vi "S_curve_scan.vi"() -> ()   [LabVIEW 2017]
panel:
  out "Array 3":dbl[](array[numeric])=[0.064, 0.08600000000000001, 0.10600000000000001, 0.126, 0.14600000000000002, 0.168]
  out "Array 2":dbl[](array[numeric])=[-0.03, -0.04, -0.05, -0.06, -0.07, -0.08]
  out "XY Graph 2":cluster{dbl[], dbl[]}(graph)={[-0.03, -0.04, -0.05, -0.06, -0.07, -0.08], [0.064, 0.08600000000000001, 0.10600000000000001, 0.126, 0.14600000000000002, 0.168]}
  out "time":dbl=10.00580883026123
  out "Current Input":dbl=-0.2
  out "Current DC":dbl=-0.08
  in  "DC end":dbl=-0.08
  in  "DC step":dbl=-0.01
  in  "DC start":dbl=-0.03
  out "Array":dbl[](array[numeric])=[0.05, 0.052000000000000005, 0.054000000000000006, 0.056, 0.058, 0.060000000000000005, 0.062, 0.064, 0.066, 0.068, 0.07, 0.07200000000000001, 0.07400000000000001, 0.07600000000000001, 0.078, 0.08, 0.082, 0.084, 0.08600000000000001, 0.088, 0.09, 0.092, 0.094, 0.096, 0.098, 0.1, 0.10200000000000001, 0.10400000000000001, 0.10600000000000001, 0.10800000000000001, 0.11, 0.112, 0.114, 0.116, 0.11800000000000001, 0.12000000000000001, 0.12200000000000001, 0.124, 0.126, 0.128, 0.13, 0.132, 0.134, 0.136, 0.138, 0.14, 0.14200000000000002, 0.14400000000000002, 0.14600000000000002, 0.14800000000000002, 0.15000000000000002, 0.15200000000000002, 0.15400000000000003, 0.156, 0.158, 0.16, 0.162, 0.164, 0.166, 0.168, 0.16999999999999998, 0.172, 0.174, 0.176, 0.178, 0.18, 0.182, 0.184, 0.186, 0.188, 0.19, 0.192, 0.194, 0.196, 0.198, 0.2]
  out "XY Graph":cluster{dbl[], dbl[]}[](graph)=[{[0.05, 0.052000000000000005, 0.054000000000000006, 0.056, 0.058, 0.060000000000000005, 0.062, 0.064, 0.066, 0.068, 0.07, 0.07200000000000001, 0.07400000000000001, 0.07600000000000001, 0.078, 0.08, 0.082, 0.084, 0.08600000000000001, 0.088, 0.09, 0.092, 0.094, 0.096, 0.098, 0.1, 0.10200000000000001, 0.10400000000000001, 0.10600000000000001, 0.10800000000000001, 0.11, 0.112, 0.114, 0.116, 0.11800000000000001, 0.12000000000000001, 0.12200000000000001, 0.124, 0.126, 0.128, 0.13, 0.132, 0.134, 0.136, 0.138, 0.14, 0.14200000000000002, 0.14400000000000002, 0.14600000000000002, 0.14800000000000002, 0.15000000000000002, 0.15200000000000002, 0.15400000000000003, 0.156, 0.158, 0.16, 0.162, 0.164, 0.166, 0.168, 0.16999999999999998, 0.172, 0.174, 0.176, 0.178, 0.18, 0.182, 0.184, 0.186, 0.188, 0.19, 0.192, 0.194, 0.196, 0.198, 0.2], [0.0, 0.0, 55.75732653647227, 837.2048665123053, 983.9806519584773, 1021.9354209939636, 1803.5148689143737, 4499.995708469669, 3049.525954503456, 1609.084946368664, 1051.6061837442705, 986.0555933130726, 986.0551249986939, 986.5456938600472, 996.0152777764586, 985.8093213558733, 986.8265731766209, 986.0120419788054, 985.7260100320713, 986.4032052466767, 985.9937796609445, 995.4229054084522, 986.4542901805016, 986.0808829501203, 986.3539999923987, 986.0551249986939, 986.2092244347722, 986.0246855182378, 986.5508504697589, 995.3548726375087, 985.6731286894251, 996.4080596300112, 986.3455652988566, 986.2574782315413, 986.0345196064184, 986.0499735698887, 986.6910371473991, 996.0001405792435, 986.8706655854496, 986.0560616278959, 985.3989854500167, 996.0157508212853, 987.0067201898539, 995.7991433044365, 986.0134468005078, 986.4467911432761, 995.9783816643079, 995.8166386667946, 986.0462271100196, 996.0162238665615, 995.7088391835495, 986.0551249986939, 985.4518373804069, 986.721986731739, 995.7428786041428, 995.0238181093546, 986.2373328684423, 995.9968293786845, 985.8860925693159, 985.4017916046889, 986.0555933130726, 996.1032718457116, 985.7985556172813, 986.5864794279437, 996.0143316881528, 985.8289811374509, 996.2849862135934, 987.039097327572, 996.4393061826074, 986.0368610848977, 995.8596704166589, 986.190017926578, 985.4022592986881, 986.0274952377017, 986.0799462737634, 995.4479475892159]}, {[0.05, 0.052000000000000005, 0.054000000000000006, 0.056, 0.058, 0.060000000000000005, 0.062, 0.064, 0.066, 0.068, 0.07, 0.07200000000000001, 0.07400000000000001, 0.07600000000000001, 0.078, 0.08, 0.082, 0.084, 0.08600000000000001, 0.088, 0.09, 0.092, 0.094, 0.096, 0.098, 0.1, 0.10200000000000001, 0.10400000000000001, 0.10600000000000001, 0.10800000000000001, 0.11, 0.112, 0.114, 0.116, 0.11800000000000001, 0.12000000000000001, 0.12200000000000001, 0.124, 0.126, 0.128, 0.13, 0.132, 0.134, 0.136, 0.138, 0.14, 0.14200000000000002, 0.14400000000000002, 0.14600000000000002, 0.14800000000000002, 0.15000000000000002, 0.15200000000000002, 0.15400000000000003, 0.156, 0.158, 0.16, 0.162, 0.164, 0.166, 0.168, 0.16999999999999998, 0.172, 0.174, 0.176, 0.178, 0.18, 0.182, 0.184, 0.186, 0.188, 0.19, 0.192, 0.194, 0.196, 0.198, 0.2], [0.0, 0.0, 0.0, 0.0, 0.0, 0.0, 0.0, 0.0, 0.0, 0.0, 0.0, 59.10300707380999, 739.6342326489519, 985.0749820770844, 986.0921232052048, 1029.3348611838042, 1584.158804753076, 3717.642295716618, 3828.5116463705967, 2396.1575137525797, 1655.1741866864104, 1290.6405638611882, 1022.615815900484, 996.4350451736746, 985.3924378179347, 995.9708135689169, 995.4021166306491, 986.0846296733428, 986.0560616278959, 986.0799462737634, 986.0565299431642, 986.0345196064184, 996.4047457166491, 985.3891640345236, 986.4941307276188, 996.3763416491707, 986.0560616278959, 996.7381411254197, 985.4424826435281, 996.0512304639448, 985.9858193751217, 996.1676214362394, 995.8213672486362, 986.0251538037031, 996.0247387583696, 985.8565997741654, 986.0569982588773, 986.1942339252676, 986.0555933130726, 986.2804355788264, 986.8382994964995, 986.2410807806588, 986.0190661273479, 986.0476320291343, 995.7929964311694, 986.0560616278959, 985.6211888235716, 986.571477447682, 985.1806220998183, 996.031834612756, 986.0574665750353, 996.0086551960623, 986.0289001034386, 986.5077241211532, 986.0120419788054, 995.4129833834563, 995.6459669290987, 995.4781888831611, 985.1011562544927, 985.8664305098187, 986.3460338891579, 986.0579348916381, 985.4724184267322, 985.5014204511742, 986.1848650882431, 986.7022913170617]}, {[0.05, 0.052000000000000005, 0.054000000000000006, 0.056, 0.058, 0.060000000000000005, 0.062, 0.064, 0.066, 0.068, 0.07, 0.07200000000000001, 0.07400000000000001, 0.07600000000000001, 0.078, 0.08, 0.082, 0.084, 0.08600000000000001, 0.088, 0.09, 0.092, 0.094, 0.096, 0.098, 0.1, 0.10200000000000001, 0.10400000000000001, 0.10600000000000001, 0.10800000000000001, 0.11, 0.112, 0.114, 0.116, 0.11800000000000001, 0.12000000000000001, 0.12200000000000001, 0.124, 0.126, 0.128, 0.13, 0.132, 0.134, 0.136, 0.138, 0.14, 0.14200000000000002, 0.14400000000000002, 0.14600000000000002, 0.14800000000000002, 0.15000000000000002, 0.15200000000000002, 0.15400000000000003, 0.156, 0.158, 0.16, 0.162, 0.164, 0.166, 0.168, 0.16999999999999998, 0.172, 0.174, 0.176, 0.178, 0.18, 0.182, 0.184, 0.186, 0.188, 0.19, 0.192, 0.194, 0.196, 0.198, 0.2], [0.0, 0.0, 0.0, 0.0, 0.0, 0.0, 0.0, 0.0, 0.0, 0.0, 0.0, 0.0, 0.0, 0.0, 0.0, 0.0, 0.0, 0.0, 0.0, 0.0, 398.5664431188367, 966.7665540888203, 986.0574665750353, 996.0114934340196, 986.541943632297, 1029.0936584533865, 1564.3110304340744, 2759.465778777035, 4465.509262545248, 2733.1720744015347, 2155.734328739999, 1536.9241758508463, 1388.0527633524975, 1026.6104841412396, 986.3999247436581, 986.0555933130726, 986.4542901805016, 986.0569982588773, 986.0565299431642, 985.8013640481577, 986.0555933130726, 995.4092036164387, 995.9864228916847, 986.3591545983572, 986.0555933130726, 995.8525770150901, 986.0555933130726, 986.0555933130726, 985.873452583894, 995.4970906249673, 985.872516301571, 985.9254190412377, 986.71542150615, 986.0560616278959, 996.0157508212853, 995.9008141385821, 986.0237489486415, 995.4144008034885, 986.0565299431642, 985.9755180195582, 996.0001405792435, 996.4265232651343, 986.3427537663996, 986.4542901805016, 986.4153901632147, 986.0846296733428, 986.3966442624594, 996.0162238665615, 985.9385285624262, 985.5580260931813, 986.0757312521788, 986.4299187263807, 996.0157508212853, 986.0771362553699, 985.3952439353151, 985.8650261070073]}, {[0.05, 0.052000000000000005, 0.054000000000000006, 0.056, 0.058, 0.060000000000000005, 0.062, 0.064, 0.066, 0.068, 0.07, 0.07200000000000001, 0.07400000000000001, 0.07600000000000001, 0.078, 0.08, 0.082, 0.084, 0.08600000000000001, 0.088, 0.09, 0.092, 0.094, 0.096, 0.098, 0.1, 0.10200000000000001, 0.10400000000000001, 0.10600000000000001, 0.10800000000000001, 0.11, 0.112, 0.114, 0.116, 0.11800000000000001, 0.12000000000000001, 0.12200000000000001, 0.124, 0.126, 0.128, 0.13, 0.132, 0.134, 0.136, 0.138, 0.14, 0.14200000000000002, 0.14400000000000002, 0.14600000000000002, 0.14800000000000002, 0.15000000000000002, 0.15200000000000002, 0.15400000000000003, 0.156, 0.158, 0.16, 0.162, 0.164, 0.166, 0.168, 0.16999999999999998, 0.172, 0.174, 0.176, 0.178, 0.18, 0.182, 0.184, 0.186, 0.188, 0.19, 0.192, 0.194, 0.196, 0.198, 0.2], [0.0, 0.0, 0.0, 0.0, 0.0, 0.0, 0.0, 0.0, 0.0, 0.0, 0.0, 0.0, 0.0, 0.0, 0.0, 0.0, 0.0, 0.0, 0.0, 0.0, 0.0, 0.0, 0.0, 0.0, 0.0, 0.0, 0.0, 0.0, 14.742285289291985, 565.3567009841202, 982.3957679268094, 986.0040813981044, 986.0326464316415, 986.363372043305, 986.0555933130726, 1005.4680092956914, 1434.9752490432304, 2228.3471780801215, 4447.243205944192, 3349.4604256872603, 2468.944413808887, 2013.9585622239347, 1437.5544365170463, 1120.9821022904437, 998.5701055398292, 985.9947161736093, 996.0162238665615, 996.7798312393919, 986.3404108349292, 985.4331280842539, 986.0555933130726, 985.8594085357746, 986.410234969479, 986.2429547474492, 986.521317889313, 996.042715119184, 986.4702260131822, 986.5391309801954, 996.3526728299544, 986.0579348916381, 996.4184749297997, 996.0114934340196, 986.2771558923512, 986.3891461016548, 995.5755405246308, 986.4402295792314, 986.0555933130726, 985.4555793248887, 986.0509101893043, 995.9235155784011, 986.4519467191208, 985.8987328788589, 985.8299173370851, 986.7904578623395, 986.4233573867945, 985.1665977837577]}, {[0.05, 0.052000000000000005, 0.054000000000000006, 0.056, 0.058, 0.060000000000000005, 0.062, 0.064, 0.066, 0.068, 0.07, 0.07200000000000001, 0.07400000000000001, 0.07600000000000001, 0.078, 0.08, 0.082, 0.084, 0.08600000000000001, 0.088, 0.09, 0.092, 0.094, 0.096, 0.098, 0.1, 0.10200000000000001, 0.10400000000000001, 0.10600000000000001, 0.10800000000000001, 0.11, 0.112, 0.114, 0.116, 0.11800000000000001, 0.12000000000000001, 0.12200000000000001, 0.124, 0.126, 0.128, 0.13, 0.132, 0.134, 0.136, 0.138, 0.14, 0.14200000000000002, 0.14400000000000002, 0.14600000000000002, 0.14800000000000002, 0.15000000000000002, 0.15200000000000002, 0.15400000000000003, 0.156, 0.158, 0.16, 0.162, 0.164, 0.166, 0.168, 0.16999999999999998, 0.172, 0.174, 0.176, 0.178, 0.18, 0.182, 0.184, 0.186, 0.188, 0.19, 0.192, 0.194, 0.196, 0.198, 0.2], [0.0, 0.0, 0.0, 0.0, 0.0, 0.0, 0.0, 0.0, 0.0, 0.0, 0.0, 0.0, 0.0, 0.0, 0.0, 0.0, 0.0, 0.0, 0.0, 0.0, 0.0, 0.0, 0.0, 0.0, 0.0, 0.0, 0.0, 0.0, 0.0, 0.0, 0.0, 0.0, 0.0, 0.0, 0.0, 0.0, 0.0, 59.06384218274547, 114.50487420346302, 892.8572340887513, 986.4336681024776, 986.0555933130726, 985.4668053288425, 986.0832246487978, 986.4022679578735, 1009.1791967425504, 1397.4597572462005, 2133.893863166398, 4230.0, 4013.5982293714296, 2707.2941929681488, 2446.025059984004, 1961.3663143726196, 1422.7771960409455, 1072.299897409147, 989.0110606221558, 996.8992358610527, 995.9850038421243, 996.346045762083, 986.0541883712713, 986.3872715792654, 986.0565299431642, 986.4322620831011, 986.4500719580329, 985.4682085973203, 996.349359284999, 995.6412400128564, 985.9933114052793, 985.0726451645962, 986.4467911432761, 996.3100717889857, 995.2339484480553, 986.4491345801613, 985.4022592986881, 995.4266852795275, 986.0584032086857]}, {[0.05, 0.052000000000000005, 0.054000000000000006, 0.056, 0.058, 0.060000000000000005, 0.062, 0.064, 0.066, 0.068, 0.07, 0.07200000000000001, 0.07400000000000001, 0.07600000000000001, 0.078, 0.08, 0.082, 0.084, 0.08600000000000001, 0.088, 0.09, 0.092, 0.094, 0.096, 0.098, 0.1, 0.10200000000000001, 0.10400000000000001, 0.10600000000000001, 0.10800000000000001, 0.11, 0.112, 0.114, 0.116, 0.11800000000000001, 0.12000000000000001, 0.12200000000000001, 0.124, 0.126, 0.128, 0.13, 0.132, 0.134, 0.136, 0.138, 0.14, 0.14200000000000002, 0.14400000000000002, 0.14600000000000002, 0.14800000000000002, 0.15000000000000002, 0.15200000000000002, 0.15400000000000003, 0.156, 0.158, 0.16, 0.162, 0.164, 0.166, 0.168, 0.16999999999999998, 0.172, 0.174, 0.176, 0.178, 0.18, 0.182, 0.184, 0.186, 0.188, 0.19, 0.192, 0.194, 0.196, 0.198, 0.2], [0.0, 0.0, 0.0, 0.0, 0.0, 0.0, 0.0, 0.0, 0.0, 0.0, 0.0, 0.0, 0.0, 0.0, 0.0, 0.0, 0.0, 0.0, 0.0, 0.0, 0.0, 0.0, 0.0, 0.0, 0.0, 0.0, 0.0, 0.0, 0.0, 0.0, 0.0, 0.0, 0.0, 0.0, 0.0, 0.0, 0.0, 0.0, 0.0, 0.0, 0.0, 0.0, 0.0, 0.0, 0.0, 0.0, 0.0, 226.95350262997795, 869.565345589509, 985.3798104874976, 986.4486658918935, 985.4855159038125, 985.8467692345679, 986.0555933130726, 986.463195435296, 999.3285875416535, 1339.2183669656915, 1975.030597994271, 3596.3781592024634, 4462.327140965309, 3017.00479317694, 2495.0297170023723, 2251.986487707475, 1633.467382936151, 1478.1033439166642, 1307.6598513497754, 1026.8366826174322, 986.318856387641, 986.8246969913018, 986.053251745628, 996.2731538334734, 986.4149215070122, 986.0555933130726, 985.4770960571527, 986.0715162666285, 985.9581934978955]}]
  out "Waveform Graph":dbl[](graph)=[0.0, 0.0, 0.0, 0.0, 0.0, 0.0, 0.0, 0.0, 0.0, 0.0, 0.0, 0.0, 0.0, 0.0, 0.0, 0.0, 0.0, 0.0, 0.0, 0.0, 0.0, 0.0, 0.0, 0.0, 0.0, 0.0, 0.0, 0.0, 0.0, 0.0, 0.0, 0.0, 0.0, 0.0, 0.0, 0.0, 0.0, 0.0, 0.0, 0.0, 0.0, 0.0, 0.0, 0.0, 0.0, 0.0, 0.0, 226.95350262997795, 869.565345589509, 985.3798104874976, 986.4486658918935, 985.4855159038125, 985.8467692345679, 986.0555933130726, 986.463195435296, 999.3285875416535, 1339.2183669656915, 1975.030597994271, 3596.3781592024634, 4462.327140965309, 3017.00479317694, 2495.0297170023723, 2251.986487707475, 1633.467382936151, 1478.1033439166642, 1307.6598513497754, 1026.8366826174322, 986.318856387641, 986.8246969913018, 986.053251745628, 996.2731538334734, 986.4149215070122, 986.0555933130726, 985.4770960571527, 986.0715162666285, 985.9581934978955]
  in  "input end":dbl=-0.2
  in  "input step":dbl=-0.002
  in  "input start":dbl=-0.05
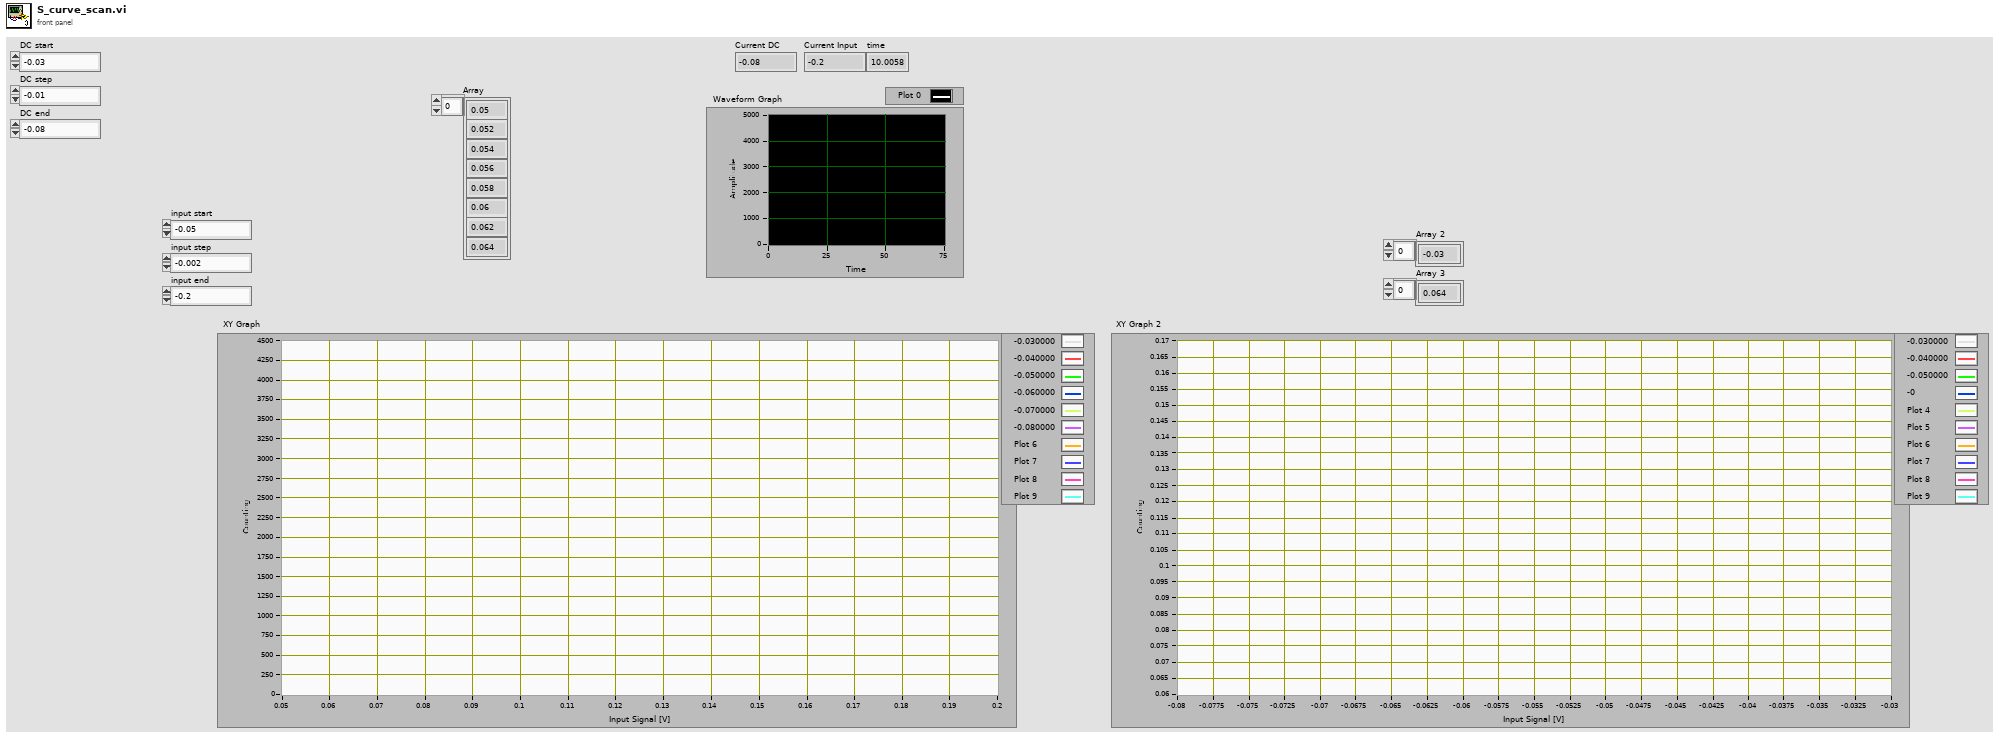
[diagram p1: front panel]
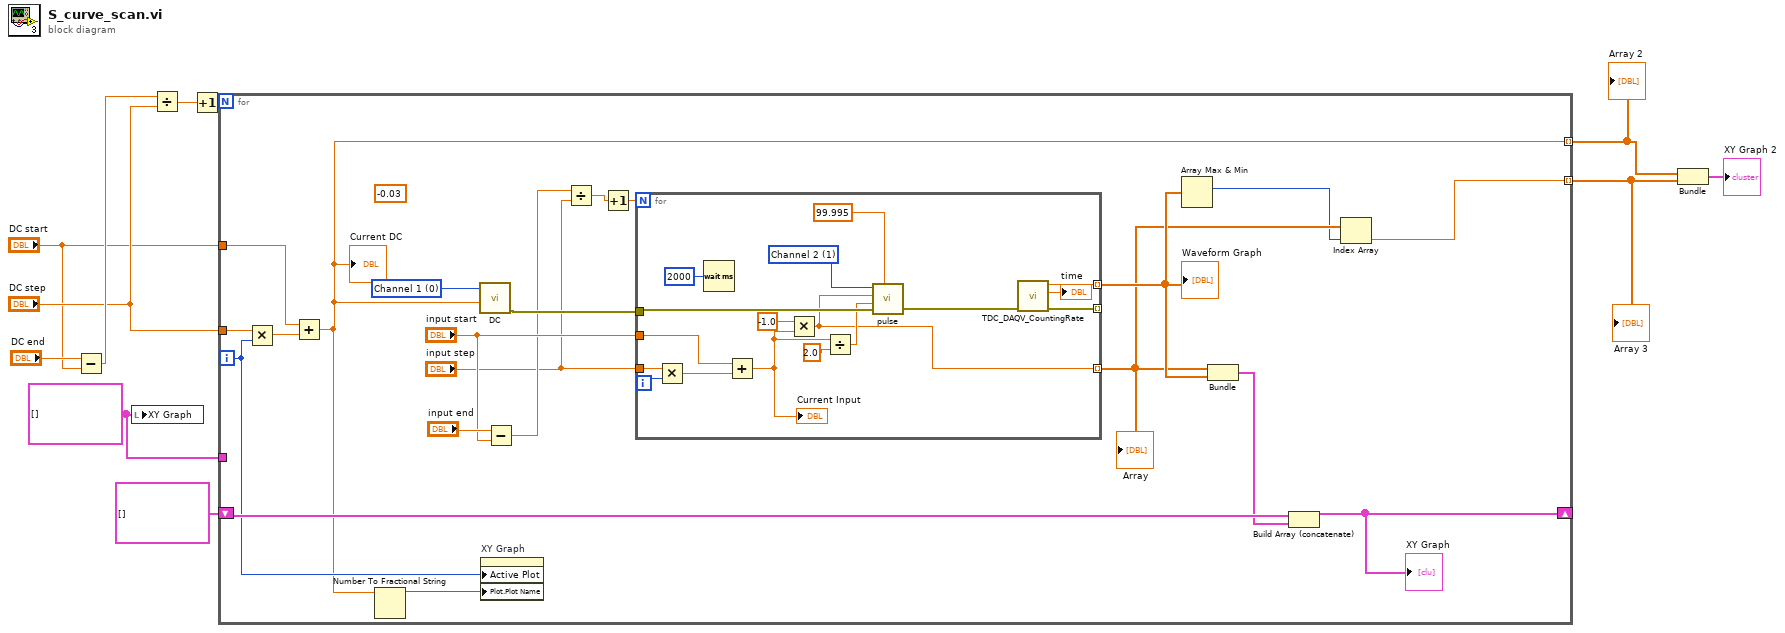
[diagram p0: block diagram]
diagram:
  w4 = cluster{dbl[], dbl[]}[] [] ("XY Graph")
  n1 = Subtract(x="DC end", y="DC start") -> (x-y=w8:dbl)
  n2 = local write "XY Graph"(w4) -> ()
  n3 = Divide(x=w8, y="DC step") -> (x/y=w10:dbl)
  n4 = Increment(x=w10) -> (x+1=w11:dbl)
  n5 = for {
    N: w11 -> [_]
    tunnel: "DC step" -> [w24]
    tunnel: "DC start" -> [w22]
    shift-right: [w19] -> _
    shift-left: cluster{dbl[], dbl[]}[] [] -> [w21]
    tunnel: w4 -> [_]
    tunnel: [w12] -> w2 mode=indexing
    tunnel: [w15] -> w3 mode=indexing
    i -> [w18]
    (unwired) -0.03 ("DC Offset (0.00 V)")
    w32 = u16 0 items=["Channel 1", "Channel 2"] ("Channel (0: Channel 1)")
    n6 = Multiply(x=w24, y=w18) -> (x*y=w23:dbl)
    n7 = Add(x=w22, y=w23) -> (x+y=w15:dbl)
    "Current DC" <- w15
    n8 = Number To Fractional String(number=w15) -> (F-format string=w17:string)  [unwired: 3 in]
    n9 = call "DC.vi"("DC Offset (0.00 V)"=w15, "Channel (0: Channel 1)"=w32) -> ("error out"=w31:errorcluster)  [unwired: 9 in]
    n10 = property on="XY Graph" class="XYGraph (strict)"("Active Plot"=w18, "Plot.Plot Name"=w17) -> ()  [unwired: 2 in, 2 out]
    n11 = Subtract(x="input end", y="input start") -> (x-y=w28:dbl)
    n12 = Divide(x=w28, y="input step") -> (x/y=w26:dbl)
    n13 = Increment(x=w26) -> (x+1=w25:dbl)
    n14 = for {
      N: w25 -> [_]
      tunnel: w31 -> [w48]
      tunnel: "input start" -> [w44]
      tunnel: "input step" -> [w47]
      tunnel: [w42] -> _ mode=indexing
      tunnel: [w41] -> w16 mode=indexing
      tunnel: [w36] -> w14 mode=indexing
      i -> [w46]
      w49 = u16 1 items=["Channel 1", "Channel 2"] ("Channel (0: Channel 1)")
      n15 = Multiply(x=w47, y=w46) -> (x*y=w45:dbl)
      n16 = Wait (ms)(milliseconds to wait=u32 2000) -> ()  [unwired: 1 out]
      n17 = Add(x=w44, y=w45) -> (x+y=w37:dbl)
      "Current Input" <- w37
      n18 = Multiply(x=-1.0, y=w37) -> (x*y=w36:dbl)
      n19 = Divide(x=w37, y=2.0) -> (x/y=w39:dbl)
      n20 = call "pulse.vi"("Duty Cycle (50%)"=99.995, "error in (no error)"=w48, "DC Offset (0.00 V)"=w39, "Amplitude (1 Vpp)"=w36, "Channel (0: Channel 1)"=w49) -> ("error out"=w43:errorcluster)  [unwired: 6 in]
      n21 = call "TDC_DAQV_CountingRate.vi"("error in (no error)"=w43) -> ("error out"=w42:errorcluster, "time"=→"time":dbl, "rate"=w41:dbl)  [unwired: 8 in]
    }
    "Waveform Graph" <- w16
    "Array" <- w14
    n22 = Array Max & Min(array=w16) -> (max index (indices)=w13:i32)  [unwired: 3 out]
    n23 = Bundle(w14, w16) -> (w20:cluster{dbl[], dbl[]})  [unwired: 1 in]
    n24 = Build Array (concatenate)(w21, w20) -> (w19:cluster{dbl[], dbl[]}[])
    "XY Graph" <- w19
    n25 = Index Array(array=w14, index=w13) -> (element=w12:dbl)
  }
  "Array 2" <- w3
  "Array 3" <- w2
  n26 = Bundle(w3, w2) -> (→"XY Graph 2":cluster{dbl[], dbl[]})  [unwired: 1 in]
